vi "Gauss-Seidel Iteration (rel residual).vi"(4 "max. iters":i32=10000, 5 "res. tol":dbl=1e-05, 6 "B":dbl[](array[numeric])=[6.0, 25.0, -11.0, 15.0], 7 "A":dbl[][](array[numeric])=[[10.0, -1.0, 2.0, 0.0], [-1.0, 11.0, -1.0, 3.0], [2.0, -1.0, 10.0, -1.0], [0.0, 3.0, -1.0, 8.0]]) -> (0 "Converged?":bool=TRUE, 1 "Iterations":i32=10, 3 "X":dbl[](array[numeric])=[1.0, 2.0, -1.0, 1.0])   [LabVIEW 2017]
panel:
  in  "Stop":bool
  out "Residual":sgl(graph)
  # "PN 21/10/17"
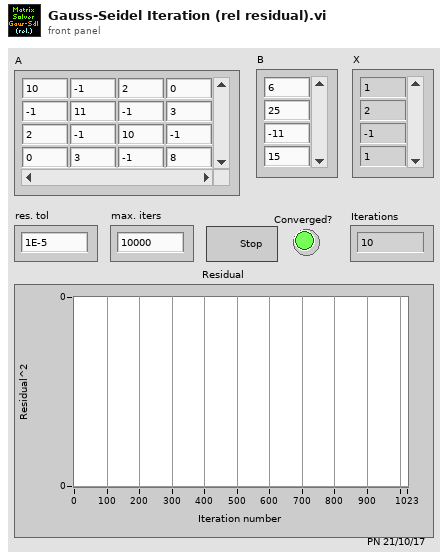
[diagram p1: front panel]
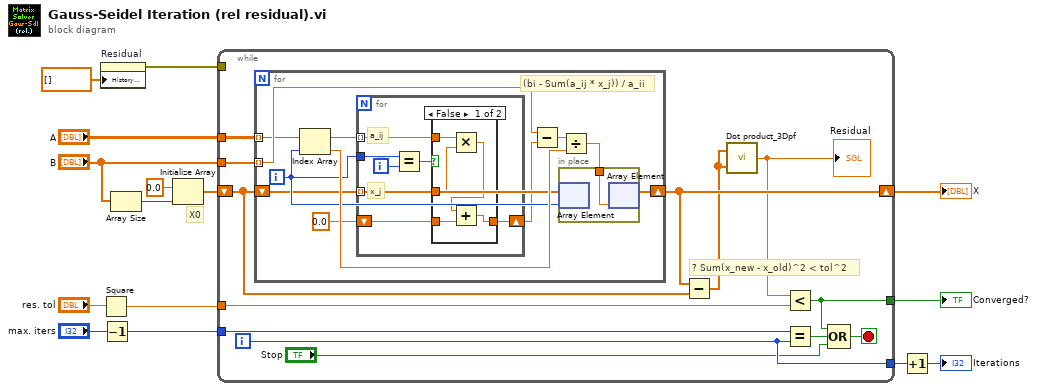
[diagram p0: block diagram]
diagram:
  # "X0"
  n1 = property on="Residual" class="WFChart (strict)"("History Data"=sgl[] []) -> (error out=w3:errorcluster)  [unwired: 2 in, 1 out]
  n2 = Square(x="res. tol") -> (x^2=w2:dbl)
  n3 = Decrement(x="max. iters") -> (x-1=w10:i32)
  n4 = Array Size(array="B") -> (size(s)=w14:i32)
  n5 = Initialize Array(0.0 ("element"), w14) -> (w13:dbl[])
  n6 = while {
    tunnel: "A" -> [w28]
    tunnel: "B" -> [w27]
    tunnel: w2 -> [w25]
    shift-right: [w21] -> w6
    shift-left: w13 -> [w26]
    tunnel: w10 -> [w23]
    tunnel: [w22] -> w9
    tunnel: w3 -> [_]
    tunnel: [w17] -> w1
    i -> [w22]
    stop <- w24 stop-if-true
    # "? Sum(x_new - x_old)^2 < tol^2"
    n7 = for {
      tunnel: w27 -> [w38] mode=indexing
      tunnel: w28 -> [w35] mode=indexing
      shift-right: [w31] -> w21
      shift-left: w26 -> [w33]
      i -> [w34]
      # "(bi - Sum(a_ij * x_j)) / a_ii"
      n8 = Index Array(array=w35, index=w34) -> (element=w36:dbl)
      n9 = for {
        tunnel: w34 -> [w44]
        tunnel: w35 -> [w42] mode=indexing
        tunnel: w33 -> [w41] mode=indexing
        shift-right: [w40] -> w29
        shift-left: 0.0 ("element") -> [w39]
        i -> [w45]
        # "x_j"
        # "a_ij"
        # "j"
        n10 = Equal?(x=w44, y=w45) -> (x = y?=w43:bool)
        n11 = case shown="False" w43 {
          tunnel: w42 -> [w50 _]
          tunnel: w41 -> [w49 _]
          tunnel: [w48 w51] -> w40
          tunnel: w39 -> [w47 w51]
          frame False {
            n12 = Multiply(x=w50, y=w49) -> (x*y=w46:dbl)
            n13 = Add(x=w46, y=w47) -> (x+y=w48:dbl)
          }
          frame True {
          }
        }
      }
      n14 = Subtract(x=w38, y=w29) -> (x-y=w37:dbl)
      n15 = Divide(x=w37, y=w36) -> (x/y=w32:dbl)
      n16 = in-place {
        in-place-border: w32 -> [w52]
        n17 = in-place-array #1(w33, w34) -> ()  [unwired: 1 out]
        n18 = in-place-array #1(w52) -> (w31:dbl[])  [unwired: 1 out]
      }
    }
    n19 = Subtract(x=w21, y=w26) -> (x-y=w20:dbl[])
    n20 = call "Dot product_3Dpf.vi"("B"=w20, "A"=w20) -> ("A . B"=w19:sgl)
    "Residual" <- w19
    n21 = Less?(x=w19, y=w25) -> (x < y?=w17:bool)
    n22 = Equal?(x=w23, y=w22) -> (x = y?=w18:bool)
    n23 = Compound Arithmetic op=OR(w17, w18, "Stop") -> (w24:bool)
  }
  "X" <- w6
  "Converged?" <- w1
  n24 = Increment(x=w9) -> (x+1=→"Iterations":i32)
